vi "实验3-3.vi"() -> ()   [LabVIEW 2018]
panel:
  in  "输入完成":bool
  out "时间(s)":dbl
  in  "输出":string="A virtual instrument is a program in the graphical programming language."
  in  "输入":string="A virtual instrument is a program in the graphical programming language."
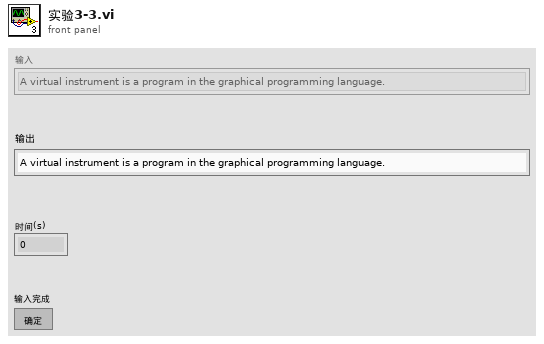
[diagram p1: front panel]
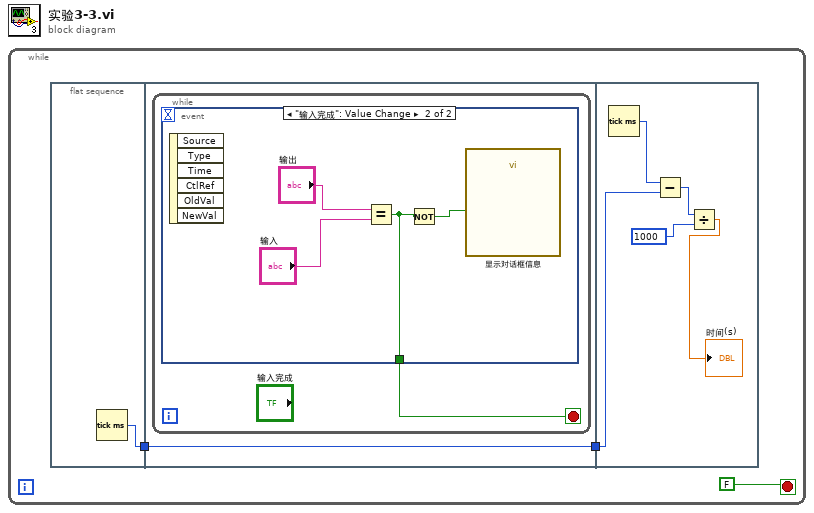
[diagram p0: block diagram]
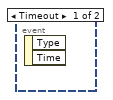
[diagram p2: hidden frame]
diagram:
  n1 = while {
    stop <- FALSE stop-if-true
    n2 = flat-sequence {
      tunnel: [w4] -> w3
      tunnel: [w5] -> w2
      tunnel: w3 -> [w5]
      tunnel: w2 -> [w14]
      frame #0 {
        n3 = Tick Count (ms)() -> (millisecond timer value=w4:u32)
      }
      frame #1 {
        n4 = while {
          stop <- w6 stop-if-true
          n5 = event shown="[1] \"输入完成\": Value Change" {
            selector: _ -> [_ _]
            dyn-events: _ -> [_ _]
            timeout: _ -> [_ _]
            tunnel: [_ w8] -> w6
            event Timeout {
              n6 = event-data() -> ()  [unwired: 1 in, 2 out]
            }
            event "输入完成": Value Change {
              n7 = event-data() -> ()  [unwired: 1 in, 6 out]
              n8 = Equal?(x="输出", y="输入") -> (x = y?=w8:bool)
              n9 = Not(x=w8) -> (.not. x?=w7:bool)
              n10 = call "显示对话框信息"("Enable"=w7) -> ()  [unwired: 9 in, 2 out]
            }
          }
        }
      }
      frame #2 {
        n11 = Tick Count (ms)() -> (millisecond timer value=w15:u32)
        n12 = Subtract(x=w15, y=w14) -> (x-y=w13:u32)
        n13 = Divide(x=w13, y=1000) -> (x/y=→"时间(s)":dbl)
      }
    }
  }
